vi "Anritsu_MT8852B_YYLL_ShowMsg.vi"(11 "reference out":refnum<vi>) -> ()   [LabVIEW 2017]
uses:
  <vilib>/Utility/miscctls.llb/LVPointTypeDef.ctl
panel:
  out "Show":string
  # "MT8852B"
  # "Anritsu"
  # "YYLL"
  # "MT8852B"
  # "Anritsu"
  # "YYLL"
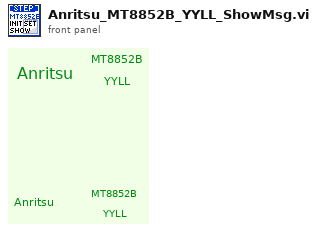
[diagram p1: front panel]
types:
  T1 = typedef "LVPointTypeDef.ctl" = cluster{"Horizontal":i16, "Vertical":i16}
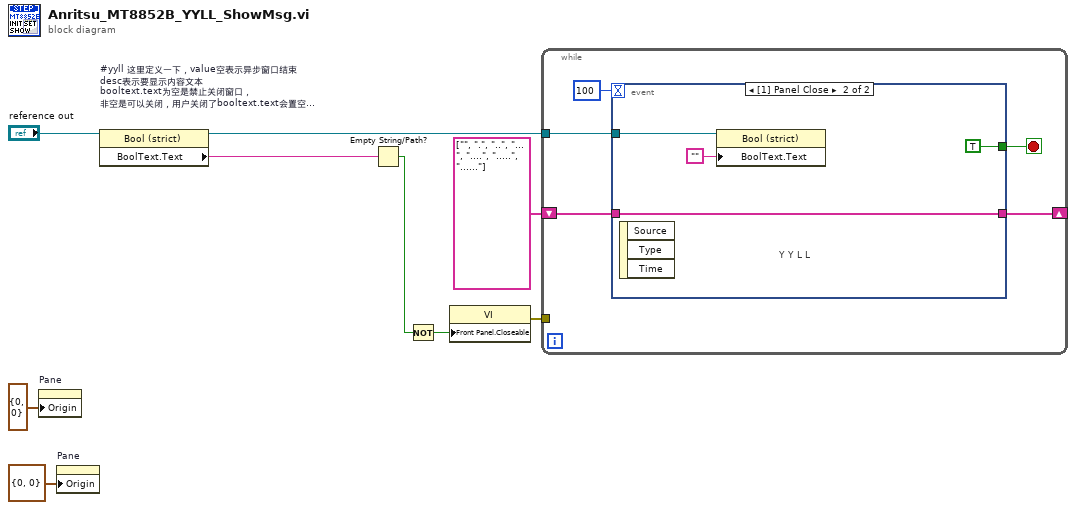
[diagram p0: block diagram]
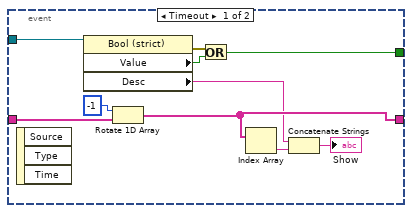
[diagram p2: hidden frame]
diagram:
  n1 = property on="Pane" class="Pane"("Origin"=T1 {"Horizontal"=0, "Vertical"=0}) -> ()  [unwired: 2 in, 2 out]
  n2 = property on="Pane" class="Pane"("Origin"=T1 {"Horizontal"=0, "Vertical"=0}) -> ()  [unwired: 2 in, 2 out]
  n3 = property on="#yyll 这里定义一下，value空表示异步窗口结束\ndesc表示要显示内容文本\nbooltext.text为空是禁止关闭窗口，\n非空是可以关闭，用户关闭了booltext.text会置空\n告知调用者表示用户手动停止了！" class="Bool (strict)"(reference="reference out") -> (reference out=w7:refnum<vi>, "BoolText.Text"=w5:string)  [unwired: 1 in, 1 out]
  n4 = Empty String/Path?(string/path=w5) -> (empty?=w4:bool)
  n5 = Not(x=w4) -> (.not. x?=w3:bool)
  n6 = property class="VI"("Front Panel.Closeable"=w3) -> (error out=w1:errorcluster)  [unwired: 2 in, 1 out]
  n7 = while {
    tunnel: w7 -> [w14]
    shift-right: [w12] -> _
    shift-left: string[] ["", ".", "..", "...", "....", ".....", "......"] ("Array") -> [w13]
    tunnel: w1 -> [_]
    stop <- w11 stop-if-true
    n8 = event shown="[1] Panel Close" {
      selector: _ -> [_ _]
      dyn-events: _ -> [_ _]
      timeout: u32 100 ("milliseconds to wait") -> [_ _]
      tunnel: w14 -> [w23 w26]
      tunnel: w13 -> [w22 w27]
      tunnel: [w20 w27] -> w12
      tunnel: [w18 TRUE] -> w11
      event Timeout {
        n9 = event-data() -> ()  [unwired: 1 in, 3 out]
        n10 = property on="Property Node" class="Bool (strict)"(reference=w23) -> (error out=w17:errorcluster, "Value"=w24:bool, "Desc"=w15:string)  [unwired: 1 in, 1 out]
        n11 = Rotate 1D Array(1:w22, 2:-1 ("n")) -> (0:w20:string[])
        n12 = Or(x=w17, y=w24) -> (x .or. y?=w18:bool)
        n13 = Index Array(array=w20) -> (element=w19:string)  [unwired: 1 in]
        n14 = Concatenate Strings(w15, w19) -> (→"Show":string)
      }
      event Panel Close {
        # "Y Y L L"
        n15 = event-data() -> ()  [unwired: 1 in, 3 out]
        n16 = property on="Property Node" class="Bool (strict)"(reference=w26, "BoolText.Text"="") -> ()  [unwired: 1 in, 2 out]
      }
    }
  }
